vi "Run.vi"(8 "error in (no error)":errorcluster, 11 "Channel Req in":refnum<class "Channel Req.lvclass">) -> (0 "error out":errorcluster, 3 "Channel Req out":refnum<class "Channel Req.lvclass">)   [LabVIEW 2018, in "Channel Req.lvclass"]
uses:
  Channel Req.lvclass
  State Machine/State Machine.lvclass
  Socket/Socket.lvclass
  RxTx/RxTx.lvclass
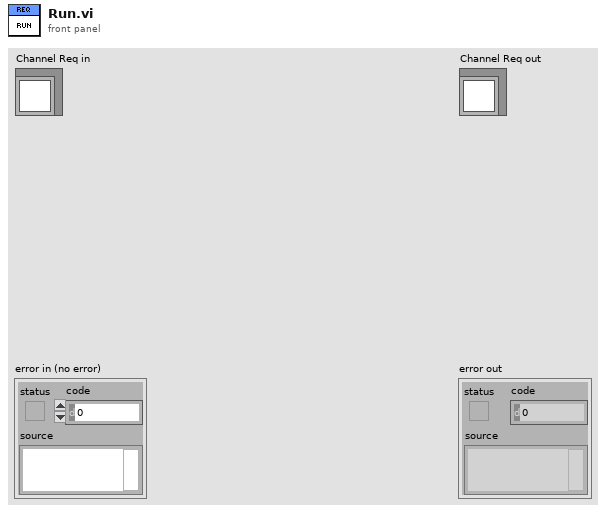
[diagram p1: front panel]
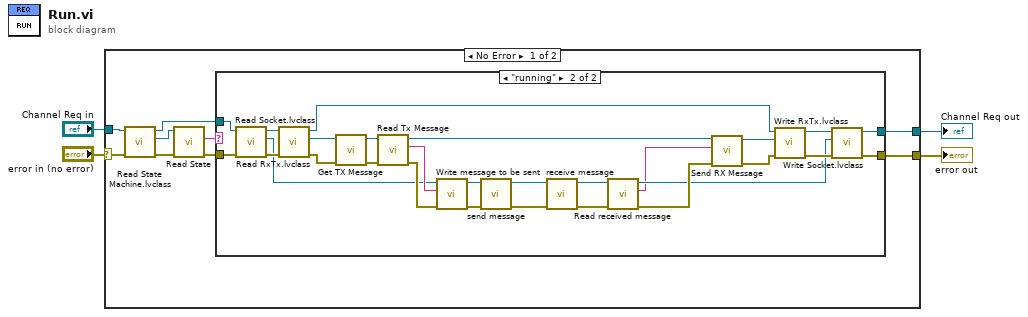
[diagram p0: block diagram]
diagram:
  n1 = case shown="No Error" "error in (no error)" {
    selector: "error in (no error)" -> [w12 w44]
    tunnel: "Channel Req in" -> [w13 w45]
    tunnel: [w6 w45] -> w2
    tunnel: [w7 w44] -> w1
    frame No Error {
      n2 = call-dynamic "Read State Machine.lvclass.vi"("error in (no error)"=w12, "Communication Channel in"=w13) -> ("error out"=w11:errorcluster, "State Machine.lvclass"=w8:refnum<class "State Machine.lvclass">, "Communication Channel out"=w9:refnum<class "Channel Req.lvclass">)  [unwired: 7 in]
      n3 = call-dynamic "Read State.vi"("error in (no error)"=w11, "State Machine in"=w8) -> ("error out"=w5:errorcluster, "State"=w10:string)  [unwired: 7 in, 1 out]
      n4 = case shown="\"running\"" w10 {
        tunnel: w9 -> [w15 w43]
        tunnel: [w15 w39] -> w6
        tunnel: [w14 w37] -> w7
        tunnel: w5 -> [w14 w36]
        frame Default {
        }
        frame "running" {
          n5 = call-dynamic "Read Socket.lvclass.vi"("error in (no error)"=w36, "Communication Channel in"=w43) -> ("error out"=w41:errorcluster, "Socket.lvclass"=w20:refnum<class "Socket.lvclass">, "Communication Channel out"=w42:refnum<class "Channel Req.lvclass">)  [unwired: 7 in]
          n6 = call-dynamic "Read RxTx.lvclass.vi"("error in (no error)"=w41, "Communication Channel in"=w42) -> ("error out"=w21:errorcluster, "RxTx.lvclass"=w22:refnum<class "RxTx.lvclass">, "Communication Channel out"=w35:refnum<class "Channel Req.lvclass">)  [unwired: 7 in]
          n7 = call "Get TX Message.vi"("error in (no error)"=w21, "RxTx in"=w22) -> ("error out"=w28:errorcluster, "RxTx out"=w27:refnum<class "RxTx.lvclass">)  [unwired: 8 in]
          n8 = call "Read Tx Message.vi"("error in (no error)"=w28, "RxTx in"=w27) -> ("error out"=w25:errorcluster, "Tx Message"=w26:string, "RxTx out"=w24:refnum<class "RxTx.lvclass">)  [unwired: 7 in]
          n9 = call-dynamic "Write message to be sent.vi"("error in (no error)"=w25, "message to be sent"=w26, "Socket in"=w20) -> ("error out"=w32:errorcluster, "Socket out"=w34:refnum<class "Socket.lvclass">)  [unwired: 7 in]
          n10 = call "send message.vi"("error in (no error)"=w32, "Socket in"=w34) -> ("error out"=w31:errorcluster, "Socket out"=w33:refnum<class "Socket.lvclass">)  [unwired: 8 in]
          n11 = call-dynamic "receive message.vi"("error in (no error)"=w31, "Socket in"=w33) -> ("error out"=w29:errorcluster, "Socket out"=w30:refnum<class "Socket.lvclass">)  [unwired: 8 in]
          n12 = call-dynamic "Read received message.vi"("error in (no error)"=w29, "Socket in"=w30) -> ("error out"=w23:errorcluster, "received message"=w16:string, "Socket out"=w17:refnum<class "Socket.lvclass">)  [unwired: 7 in]
          n13 = call "Send RX Message.vi"("error in (no error)"=w23, "message"=w16, "RxTx in"=w24) -> ("error out"=w18:errorcluster, "RxTx out"=w19:refnum<class "RxTx.lvclass">)  [unwired: 7 in]
          n14 = call-dynamic "Write RxTx.lvclass.vi"("error in (no error)"=w18, "RxTx.lvclass"=w19, "Communication Channel in"=w35) -> ("error out"=w38:errorcluster, "Communication Channel out"=w40:refnum<class "Channel Req.lvclass">)  [unwired: 7 in]
          n15 = call-dynamic "Write Socket.lvclass.vi"("error in (no error)"=w38, "Socket2.lvclass"=w17, "Communication Channel in"=w40) -> ("error out"=w37:errorcluster, "Communication Channel out"=w39:refnum<class "Channel Req.lvclass">)  [unwired: 7 in]
        }
      }
    }
    frame Error {
    }
  }
  "error out" <- w1
  "Channel Req out" <- w2
